vi "Post-Build Action_SrcDist.vi"(5 "Files Generated by Build":path[](array[path]), 6 "Top Level/Always Included VIs":path[](array[path]), 7 "Destination Path":path, 8 "error in (no error)":errorcluster, 9 "Target Name":string, 10 "Build Specification Name":string, 11 "Project Path":path) -> (0 "error out":errorcluster)   [LabVIEW 2017, in "NIPKG_VIComponentBuilder_BuildSteps.lvlib"]
doc: "<B>Package details</B>\nVI Component Builder - NIPKG - v1.0.0-21\n\nPackage Filename - vicomponentbuilder-nipkg-1.0.0-21.nipkg"
uses:
  NIPKG_VIComponentBuilder_BuildSteps.lvlib
  Source/CL_G3_VIComponentBuilder.lvlib
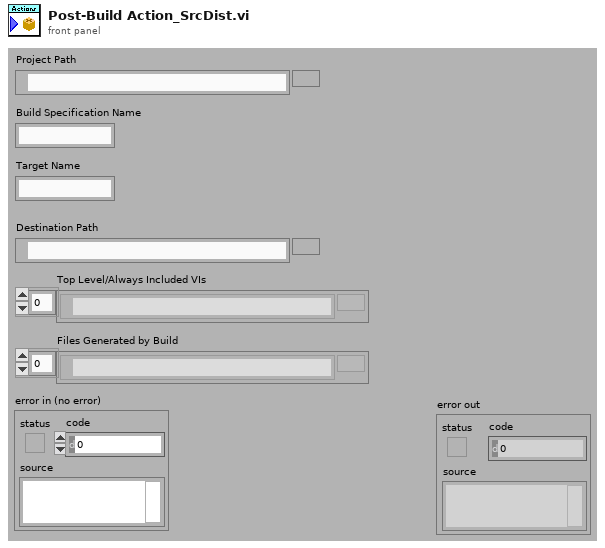
[diagram p1: front panel]
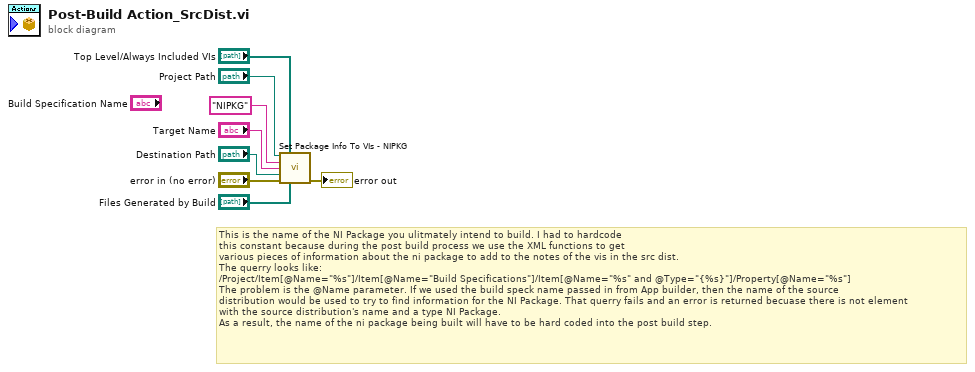
[diagram p0: block diagram]
diagram:
  # "This is the name of the NI Package you ulitmately intend to build. I had to hardcode\nthis constant because during the post build process we use the XML functions to get\nvarious pieces of information about the ni package to add to the notes of the vis in the src dist.\nThe querry looks like:\n/Project/Item[@Name=\"%s\"]/Item[@Name=\"Build Specifications\"]/Item[@Name=\"%s\" and @Type=\"{%s}\"]/Property[@Name=\"%s\"]\nThe problem is the @Name parameter. If we used the build speck name passed in from App builder, then the name of the source\ndistribution would be used to try to find information for the NI Package. That querry fails and an error is returned becuase there is not element\nwith the source distribution's name and a type NI Package. \nAs a result, the name of the ni package being built will have to be hard coded into the post build step."
  n1 = call "Set Package Info To VIs - NIPKG.vi"("Project Path"="Project Path", "Top Level/Always Included VIs"="Top Level/Always Included VIs", "NIPKG Build Spec Name (NIPKG)"="NIPKG", "Target Name (My Computer)"="Target Name", "Destination Path"="Destination Path", "error in"="error in (no error)", "Files Generated By Build"="Files Generated by Build") -> ("error out"=→"error out":errorcluster)  [unwired: 8 in]
